vi "DAQ.vi"   [LabVIEW 2015]
uses:
  Controls/Channel Configuration.ctl
  CAN Communication/Gas/Typedefs/Session Handle.ctl
  CAN Communication/Gas/Gas.lvclass
  CAN Communication/Peltier/Typedefs/Session Handle.ctl
  CAN Communication/Peltier/Peltier.lvclass
  Common/Buffers/Snapshot/Typedefs/Session Handle.ctl
  Common/Buffers/Snapshot/Snapshot.lvclass
  Common/Circular Error Log/Typedefs/Session Handle.ctl
  Common/Circular Error Log/Circular Error Log.lvclass
  Config/User Configuration.ctl
  Common/State Machine/State Machine.lvlib
  User Interface/UI Handler/UI Handler.lvclass
panel:
  # "DAQ"
types:
  T1 = typedef "Channel Configuration.ctl" = cluster{"Index":u16, "Name":string, "Units":string, "Gain":dbl, "Offset":dbl, "Source":string}
  T2 = typedef "Gas.lvclass/Session Handle.ctl" = refnum<data-value>
  T3 = typedef "Peltier.lvclass/Session Handle.ctl" = refnum<data-value>
  T4 = typedef "Snapshot.lvclass/Session Handle.ctl" = refnum<data-value>
  T5 = typedef "Circular Error Log.lvclass/Session Handle.ctl" = refnum<data-value>
  T6 = typedef "User Configuration.ctl" = cluster{"Password":string, "cDAQ Name":string, "CAN Interface":string}
  T7 = cluster{"State":refnum<queue>, "Root Path":path, "Channels":T1[], "Gas":T2, "Peltier":T3, "Snapshot":T4, "LogData":refnum<queue>, "Error":T5, "Alerted?":bool, "User Config":T6}
  T8 = cluster{"Averaged Values":dbl[], "seconds since 1Jan1904":timestamp}
  T9 = cluster{"Values":dbl[], "seconds since 1Jan1904":timestamp}
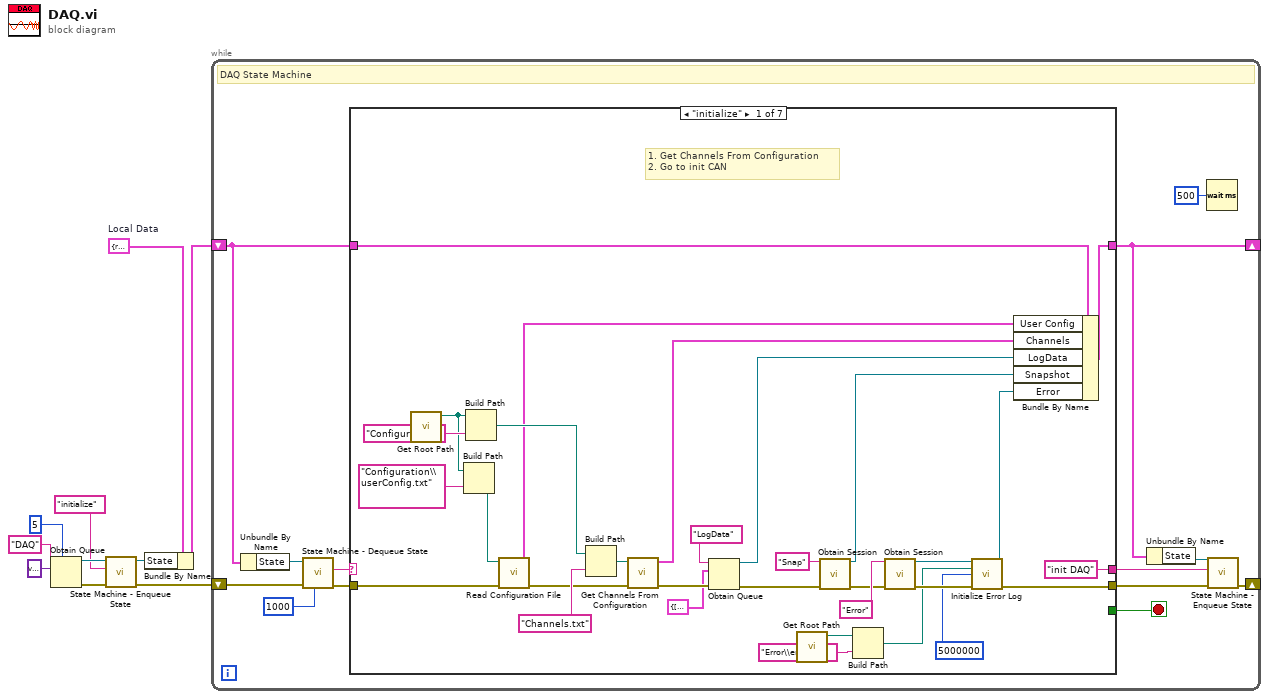
[diagram p0: block diagram]
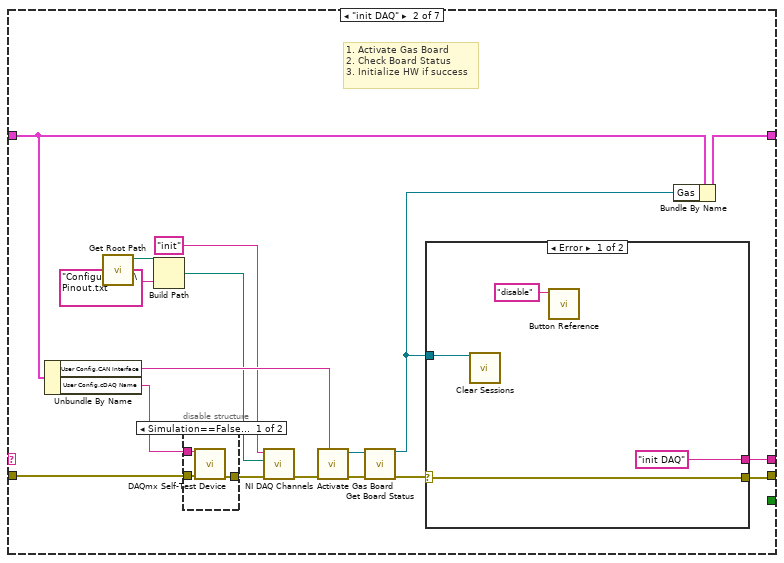
[diagram p2: hidden frame]
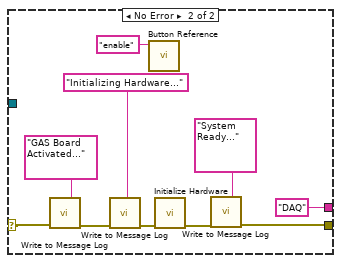
[diagram p4: hidden frame]
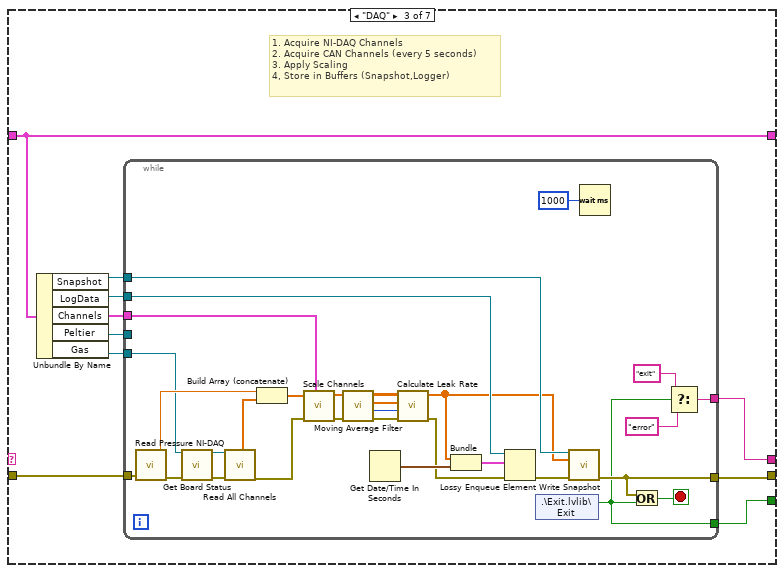
[diagram p5: hidden frame]
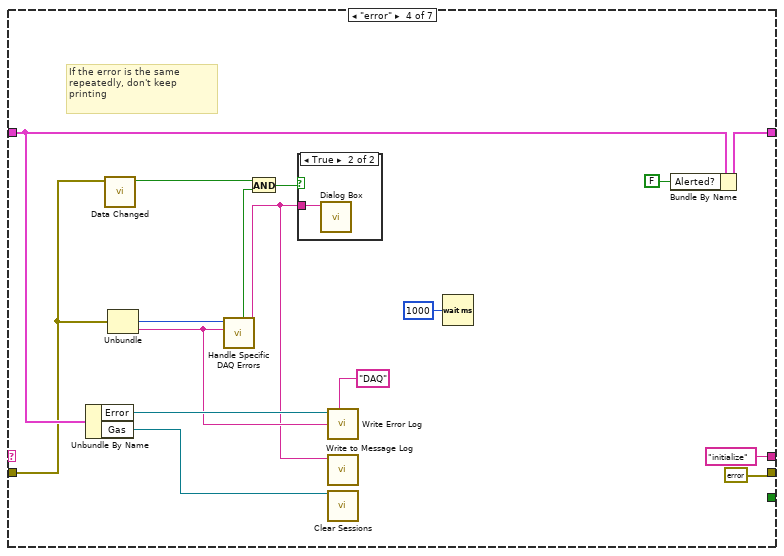
[diagram p6: hidden frame]
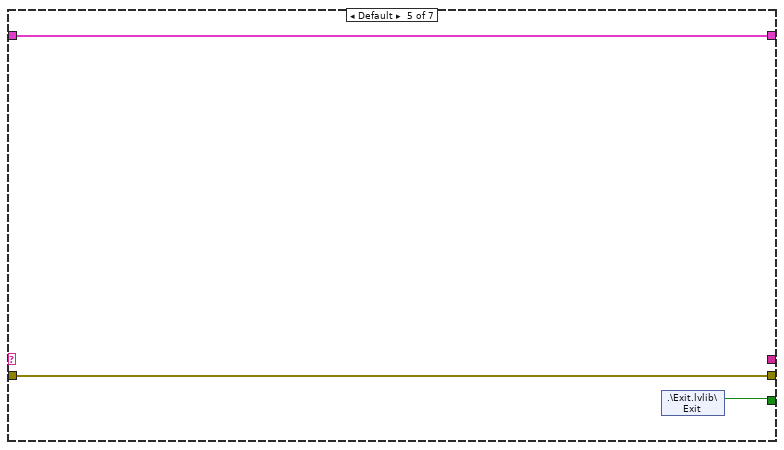
[diagram p8: hidden frame]
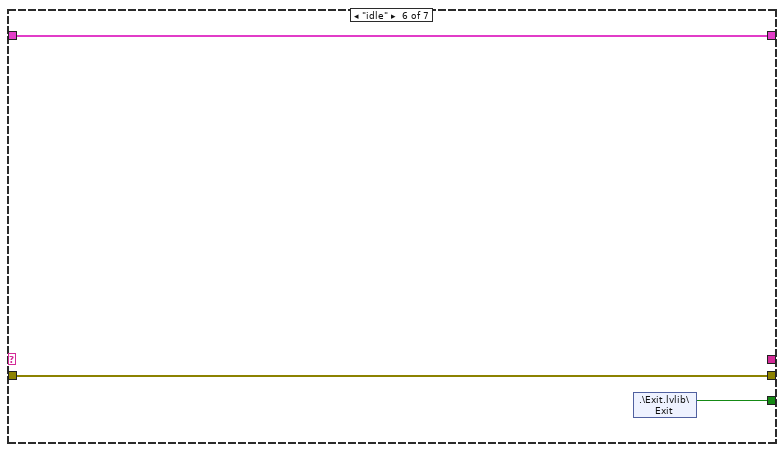
[diagram p9: hidden frame]
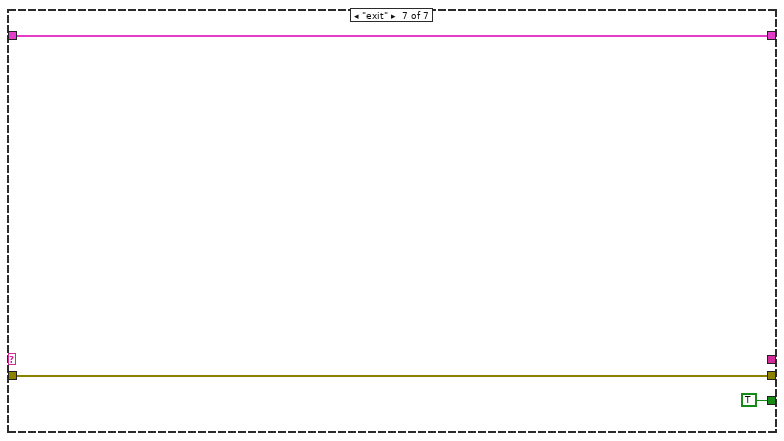
[diagram p10: hidden frame]
diagram:
  w3 = T7 {"State"=refnum, "Root Path"=path "C:/Gas Circulation Tester", "Channels"=[], "Gas"=refnum, "Peltier"=refnum, "Snapshot"=refnum, "LogData"=refnum, "Error"=refnum, "Alerted?"=FALSE, "User Config"={"Password"="", "cDAQ Name"="", "CAN Interface"=""}}  # Local Data
  n1 = Obtain Queue(max queue size (-1, unlimited)=5, name (unnamed)="DAQ", element data type=variant) -> (queue out=w6:refnum<queue>, error out=w7:errorcluster)  [unwired: 2 in, 1 out]
  n2 = call "State Machine - Enqueue State.vi"("error in (no error)"=w7, "State"="initialize", "Queue In"=w6) -> ("error out"=w4:errorcluster, "Queue Out"=w2:refnum<queue>)  [unwired: 7 in]
  n3 = Bundle By Name(cluster=w3, "State"=w2) -> (w1:T7)
  n4 = while "Main State Machine" {
    shift-right: [w20] -> _
    shift-left: w4 -> [w23]
    shift-right: [w11] -> _
    shift-left: w1 -> [w14]
    stop <- w16 stop-if-true
    # "DAQ State Machine"
    n5 = Unbundle By Name(w14) -> ("State"=w13:refnum<queue>)
    n6 = call "State Machine - Dequeue State.vi"("Timeout"=1000, "error in (no error)"=w23, "Queue In"=w13) -> ("error out"=w22:errorcluster, "State"=w21:string)  [unwired: 4 in, 3 out]
    n7 = case shown="\"initialize\"" w21 {
      tunnel: w22 -> [w32 w63 w99 w138 w149 w152 w155]
      tunnel: [w33 w69 w96 errorcluster {"status"=FALSE, "code"=0, "source"=""} ("error out") w149 w152 w155] -> w19
      tunnel: ["init DAQ" ("State") w67 w93 "initialize" ("State") _ _ _] -> w18
      tunnel: [_ _ w92 _ w147 w150 TRUE] -> w16
      tunnel: w14 -> [w50 w65 w98 w142 w148 w151 w153]
      tunnel: [w49 w71 w98 w141 w148 w151 w153] -> w11
      frame "initialize" {
        # "1. Get Channels From Configuration\n2. Go to init CAN"
        n8 = call "Get Root Path.vi"() -> ("Root Path"=w26:path)  [unwired: 11 in]
        n9 = Build Path(base path=w26, name or relative path="Configuration\\userConfig.txt") -> (appended path=w24:path)
        n10 = Build Path(base path=w26, name or relative path="Configuration") -> (appended path=w53:path)
        n11 = call "Read Configuration File.vi"("error in (no error)"=w32, "Filepath"=w24) -> ("error out"=w31:errorcluster, "User Config"=w30:T6)  [unwired: 8 in]
        n12 = Build Path(base path=w53, name or relative path="Channels.txt") -> (appended path=w51:path)
        n13 = call "Get Channels From Configuration.vi"("error in (no error)"=w31, "Path"=w51) -> ("error out"=w47:errorcluster, "Channels"=w48:T1[])  [unwired: 8 in]
        n14 = Obtain Queue(name (unnamed)="LogData", element data type=T8 {"Averaged Values"=[], "seconds since 1Jan1904"=timestamp(0 s since 1904-01-01)} ("output cluster"), error in (no error)=w47) -> (queue out=w41:refnum<queue>, error out=w45:errorcluster)  [unwired: 2 in, 1 out]
        n15 = call "Get Root Path.vi"() -> ("Root Path"=w29:path)  [unwired: 11 in]
        n16 = call "Obtain Session.vi"("Session  Name ()"="Snap", "error in (no error)"=w45) -> ("Session Handle"=w43:T4, "error out"=w35:errorcluster)  [unwired: 12 in]
        n17 = Build Path(base path=w29, name or relative path="Error\\error.txt") -> (appended path=w27:path)
        n18 = call "Obtain Session.vi"("Session  Name ()"="Error", "error in (no error)"=w35) -> ("Session Handle"=w37:T5, "error out"=w38:errorcluster)  [unwired: 12 in]
        n19 = call "Initialize Error Log.vi"("Session Handle in"=w37, "Error Path"=w27, "Max File Size"=i64 5000000, "error in (no error)"=w38) -> ("Session Handle out"=w34:T5, "error out"=w33:errorcluster)  [unwired: 10 in]
        n20 = Bundle By Name(cluster=w50, "User Config"=w30, "Channels"=w48, "LogData"=w41, "Snapshot"=w43, "Error"=w34) -> (w49:T7)
      }
      frame "init DAQ" {
        # "1. Activate Gas Board\n2. Check Board Status\n3. Initialize HW if success"
        n21 = Unbundle By Name(w65) -> ("User Config.CAN Interface"=w61:string, "User Config.cDAQ Name"=w64:string)
        n22 = call "Get Root Path.vi"() -> ("Root Path"=w60:path)  [unwired: 11 in]
        n23 = Build Path(base path=w60, name or relative path="Configuration\\Pinout.txt") -> (appended path=w56:path)
        n24 = disable-structure shown="Simulation==False, Default" {
          disable-tunnel: w63 -> [w74 w75]
          disable-tunnel: [w73 w75] -> w57
          disable-tunnel: w64 -> [w72 _]
          frame condition #0 (active) {
            n25 = call <vilib>:"DAQmx Self-Test Device.vi"("device in"=w72, "error in"=w74) -> ("error out"=w73:errorcluster)  [unwired: 13 in]
          }
          frame condition #1 {
          }
        }
        n26 = call "NI DAQ Channels.vi"("error in (no error)"=w57, "Path"=w56, "Command"="init" ("name or relative path")) -> ("error out"=w58:errorcluster)  [unwired: 7 in, 1 out]
        n27 = call "Activate Gas Board.vi"("CAN Interface"=w61, "error in (no error)"=w58) -> ("error out"=w68:errorcluster, "Session Handle out"=w70:T2)  [unwired: 8 in]
        n28 = call "Get Board Status.vi"("Session Handle in"=w70, "error in (no error)"=w68) -> ("Session Handle out"=w66:T2, "error out"=w62:errorcluster)  [unwired: 11 in, 1 out]
        n29 = case shown="Error" w62 {
          selector: w62 -> [w77 w87]
          tunnel: [w77 w81] -> w69
          tunnel: ["init DAQ" ("State") "DAQ" ("State")] -> w67
          tunnel: w66 -> [w78 _]
          frame Error {
            n30 = call "Clear Sessions.vi"("Session Handle in"=w78) -> ()  [unwired: 13 in, 2 out]
            n31 = call "Button Reference.vi"("Command"="disable") -> ()  [unwired: 10 in, 1 out]
          }
          frame No Error {
            n32 = call "Write to Message Log.vi"("error in (no error)"=w87, "Message"="GAS Board Activated...") -> ("error out"=w85:errorcluster)  [unwired: 9 in]
            n33 = call "Write to Message Log.vi"("error in (no error)"=w85, "Message"="Initializing Hardware...") -> ("error out"=w84:errorcluster)  [unwired: 9 in]
            n34 = call "Button Reference.vi"("Command"="enable") -> ()  [unwired: 10 in, 1 out]
            n35 = call "Initialize Hardware.vi"("error in"=w84) -> ("error out"=w82:errorcluster)  [unwired: 10 in]
            n36 = call "Write to Message Log.vi"("error in (no error)"=w82, "Message"="System Ready...") -> ("error out"=w81:errorcluster)  [unwired: 9 in]
          }
        }
        n37 = Bundle By Name(cluster=w65, "Gas"=w66) -> (w71:T7)
      }
      frame "DAQ" {
        # "1. Acquire NI-DAQ Channels\n2. Acquire CAN Channels (every 5 seconds)\n3. Apply Scaling\n4, Store in Buffers (Snapshot,Logger)"
        n38 = Unbundle By Name(w98) -> ("Snapshot"=w94:T4, "LogData"=w95:refnum<queue>, "Channels"=w97:T1[], "Peltier"=w90:T3, "Gas"=w91:T2)
        n39 = while {
          tunnel: w99 -> [w113]
          tunnel: w91 -> [w108]
          tunnel: w97 -> [w129]
          tunnel: [w121] -> w96
          tunnel: w95 -> [w124]
          tunnel: w94 -> [w122]
          tunnel: [w117] -> w93
          tunnel: [w116] -> w92
          tunnel: w90 -> [_]
          stop <- w125 stop-if-true
          n40 = call "Read Pressure NI-DAQ.vi"("error in (no error)"=w113) -> ("error out"=w109:errorcluster, "Pressure"=w112:dbl)  [unwired: 9 in]
          n41 = call "Get Board Status.vi"("Session Handle in"=w108, "error in (no error)"=w109) -> ("Session Handle out"=w106:T2, "error out"=w107:errorcluster)  [unwired: 11 in, 1 out]
          n42 = call "Read All Channels.vi"("error in (no error)"=w107, "Gas"=w106) -> ("error out"=w128:errorcluster, "CAN Values"=w111:dbl[])  [unwired: 8 in]
          n43 = Build Array (concatenate)(w112, w111) -> (w110:dbl[])
          n44 = call "Scale Channels.vi"("Config"=w129, "error in (no error)"=w128, "Channels In"=w110) -> ("error out"=w127:errorcluster, "Channels Out"=w126:dbl[])  [unwired: 7 in]
          n45 = call "Moving Average Filter.vi"("error in (no error)"=w127, "Values"=w126) -> ("error out"=w102:errorcluster, "Count"=w103:i32, "Averaged Values"=w104:dbl[], "Buffer"=w105:dbl[][])  [unwired: 6 in]
          n46 = Get Date/Time In Seconds() -> (seconds since 1Jan1904=w115:timestamp)
          n47 = call "Calculate Leak Rate.vi"("error in (no error)"=w102, "Count"=w103, "Averaged Values"=w104, "Buffer"=w105) -> ("error out"=w101:errorcluster, "Values"=w100:dbl[])  [unwired: 6 in]
          n48 = Bundle("Values"=w100, "seconds since 1Jan1904"=w115) -> (w114:T9)  [unwired: 1 in]
          n49 = Lossy Enqueue Element(queue=w124, element=w114, error in (no error)=w101) -> (error out=w123:errorcluster)  [unwired: 3 out]
          n50 = shared-variable ".\\Exit.lvlib\\Exit"() -> (w116:bool)  [unwired: 1 in, 1 out]
          n51 = call "Write Snapshot.vi"("Session Handle in"=w122, "Buffer"=w100, "error in (no error)"=w123) -> ("error out"=w121:errorcluster)  [unwired: 11 in, 1 out]
          n52 = Wait (ms)(milliseconds to wait=u32 1000) -> ()  [unwired: 1 out]
          n53 = Or(x=w121, y=w116) -> (x .or. y?=w125:bool)
          n54 = Select(t="exit" ("State"), s=w116, f="error" ("State")) -> (s? t:f=w117:string)
        }
      }
      frame "error" {
        # "If the error is the same repeatedly, don't keep printing"
        n55 = Unbundle By Name(w142) -> ("Error"=w143:T5, "Gas"=w131:T2)
        n56 = call "Data Changed.vi"("Data"=w138) -> ("Changed?"=w135:bool)  [unwired: 10 in]
        n57 = Unbundle(w138) -> ("code"=w139:i32, "source"=w132:string)  [unwired: 1 out]
        n58 = call "Handle Specific DAQ Errors.vi"("Error In"=w132, "code"=w139) -> ("Error Message"=w130:string, "Alert User?"=w133:bool)  [unwired: 7 in, 1 out]
        n59 = And(x=w135, y=w133) -> (x .and. y?=w134:bool)
        n60 = case shown="True" w134 {
          tunnel: w130 -> [_ w146]
          frame False {
          }
          frame True {
            n61 = call "Dialog Box.vi"("In"=w146) -> ()  [unwired: 10 in, 1 out]
          }
        }
        n62 = call "Write Error Log.vi"("Session Handle in"=w143, "Process Name"="DAQ", "Data"=w132) -> ()  [unwired: 11 in, 2 out]
        n63 = call "Write to Message Log.vi"("Message"=w130) -> ()  [unwired: 10 in, 1 out]
        n64 = call "Clear Sessions.vi"("Session Handle in"=w131) -> ()  [unwired: 13 in, 2 out]
        n65 = Wait (ms)(milliseconds to wait=u32 1000) -> ()  [unwired: 1 out]
        n66 = Bundle By Name(cluster=w142, "Alerted?"=FALSE) -> (w141:T7)
      }
      frame Default {
        n67 = shared-variable ".\\Exit.lvlib\\Exit"() -> (w147:bool)  [unwired: 1 in, 1 out]
      }
      frame "idle" {
        n68 = shared-variable ".\\Exit.lvlib\\Exit"() -> (w150:bool)  [unwired: 1 in, 1 out]
      }
      frame "exit" {
      }
    }
    n69 = Unbundle By Name(w11) -> ("State"=w12:refnum<queue>)
    n70 = Wait (ms)(milliseconds to wait=u32 500) -> ()  [unwired: 1 out]
    n71 = call "State Machine - Enqueue State.vi"("error in (no error)"=w19, "State"=w18, "Queue In"=w12) -> ("error out"=w20:errorcluster)  [unwired: 7 in, 1 out]
  }
